vi "Introspection Input.vi"(7 "DLL path":path, 8 "error in (no error)":errorcluster, 11 "session id in":i32) -> (0 "error out":errorcluster, 2 "Introspection Input":T1, 3 "session id out":i32)   [LabVIEW 2017, in "ONNX Class Library.lvlib"]
doc: "Get Input Info from ONNX"
uses:
  ONNX Class Library.lvlib
  TypeDef/IO.ctl
  TypeDef/Introspection.ctl
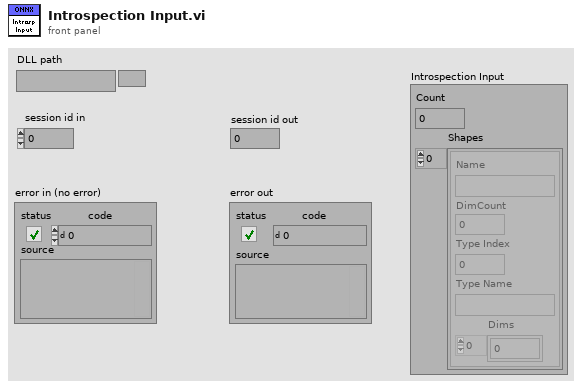
[diagram p1: front panel]
types:
  T1 = typedef "ONNX Class Library.lvlib/Introspection.ctl" = cluster{"Count":i32, "Shapes":T2[]}
  T2 = typedef "ONNX Class Library.lvlib/IO.ctl" = cluster{"Name":string, "DimCount":i32, "Type Index":i32, "Type Name":string, "Dims":i64[]}
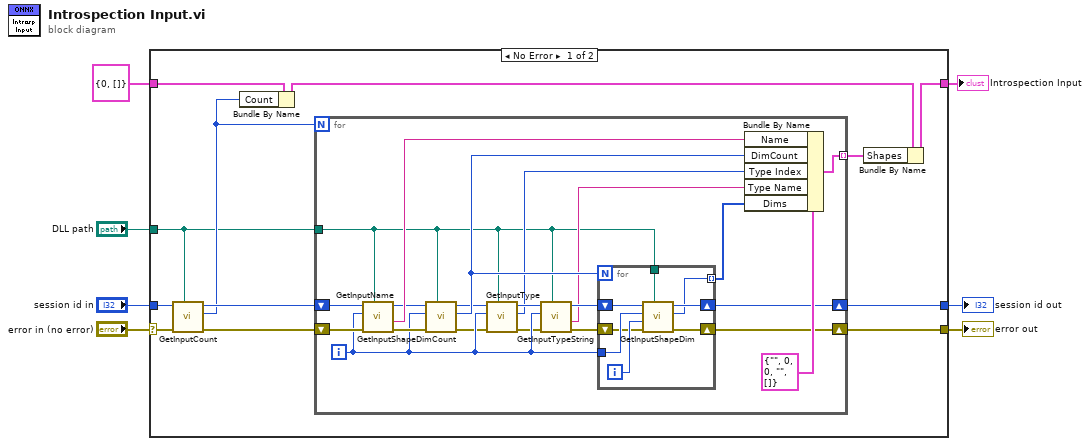
[diagram p0: block diagram]
diagram:
  n1 = case shown="No Error" "error in (no error)" {
    selector: "error in (no error)" -> [w18 w50]
    tunnel: "session id in" -> [w19 w51]
    tunnel: [w16 w51] -> w5
    tunnel: [w14 w50] -> w4
    tunnel: [w10 w49] -> w2
    tunnel: T1 {"Count"=0, "Shapes"=[]} ("Introspection") -> [w12 w49]
    tunnel: "DLL path" -> [w8 _]
    frame No Error {
      n2 = call "GetInputCount.vi"("DLL path"=w8, "error in (no error)"=w18, "session id in"=w19) -> ("error out"=w15:errorcluster, "InputCount"=w13:i32, "session id out"=w17:i32)  [unwired: 6 in]
      n3 = Bundle By Name(cluster=w12, "Count"=w13) -> (w11:T1)
      n4 = for {
        N: w13 -> [_]
        shift-right: [w24] -> w16
        shift-left: w17 -> [w40]
        shift-right: [w25] -> w14
        shift-left: w15 -> [w39]
        tunnel: [w36] -> w9 mode=indexing
        tunnel: w8 -> [w20]
        i -> [w32]
        n5 = call "GetInputName.vi"("DLL path"=w20, "error in (no error)"=w39, "index"=w32, "session id in"=w40) -> ("error out"=w34:errorcluster, "InputName"=w38:string, "session id out"=w35:i32)  [unwired: 5 in]
        n6 = call "GetInputShapeDimCount.vi"("DLL path"=w20, "error in (no error)"=w34, "inputIndex"=w32, "session id in"=w35) -> ("error out"=w29:errorcluster, "InputShapeDimCount"=w33:i32, "session id out"=w31:i32)  [unwired: 5 in]
        n7 = call "GetInputType.vi"("DLL path"=w20, "error in (no error)"=w29, "inputIndex"=w32, "session id in"=w31) -> ("error out"=w28:errorcluster, "InputTypeIndex"=w22:i32, "session id out"=w30:i32)  [unwired: 5 in]
        n8 = call "GetInputTypeString.vi"("DLL path"=w20, "error in (no error)"=w28, "input Index"=w32, "session id in"=w30) -> ("error out"=w26:errorcluster, "InputTypeName"=w21:string, "session id out"=w27:i32)  [unwired: 5 in]
        n9 = for {
          N: w33 -> [_]
          shift-right: [w44] -> w24
          shift-left: w27 -> [w45]
          shift-right: [w46] -> w25
          shift-left: w26 -> [w42]
          tunnel: w32 -> [w47]
          tunnel: [w43] -> w23 mode=indexing
          tunnel: w20 -> [w41]
          i -> [w48]
          n10 = call "GetInputShapeDim.vi"("DLL path"=w41, "error in (no error)"=w42, "dimIndex"=w48, "inputIndex"=w47, "session id in"=w45) -> ("error out"=w46:errorcluster, "InputShapeDim"=w43:i64, "session id out"=w44:i32)  [unwired: 4 in]
        }
        n11 = Bundle By Name(cluster=T2 {"Name"="", "DimCount"=0, "Type Index"=0, "Type Name"="", "Dims"=[]} ("Shape"), "Name"=w38, "DimCount"=w33, "Type Index"=w22, "Type Name"=w21, "Dims"=w23) -> (w36:T2)
      }
      n12 = Bundle By Name(cluster=w11, "Shapes"=w9) -> (w10:T1)
    }
    frame Error {
    }
  }
  "error out" <- w4
  "session id out" <- w5
  "Introspection Input" <- w2
